vi "Buffer Overflow.vi"() -> ()   [LabVIEW 2010]
uses:
  <vilib>/express/express analysis/Spectral/XNode/ExpressSpectralMeasurementsBlockNode.xnode
  Instance           2 23Saved   Buffer Overflow .vi
  Instance           5 23Saved   Buffer Overflow .vi
  Instance           4 23Saved   Buffer Overflow .vi
  <vilib>/express/express analysis/Spectral/Block/exnSpectralBlock spectral measurements power poly.vi
  <vilib>/express/express analysis/Spectral/Block/exnSpectralBlock spectral measurements power DDT.vi
  Program Files/National Instruments/LabVIEW 2010/resource/objmgr/daqmx.rc
panel:
  out "주파수":dbl
  out "파워 스펙트럼":dynamicdata(graph)
  out "시간 데이터":dynamicdata(graph)
  out "DAQ 버퍼 크기":u32
  in  "정지":bool
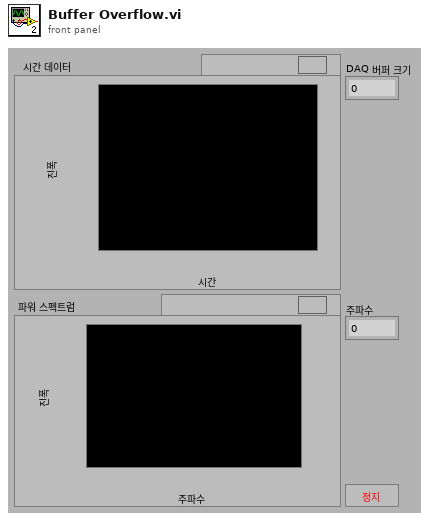
[diagram p1: front panel]
types:
  T1 = cluster{"averaging mode":u16, "weighting mode":u16, "number of averages":u32}
  T2 = cluster{"dB On (F)":bool, "unwrap phase (F)":bool, "convert to degree (F)":bool}
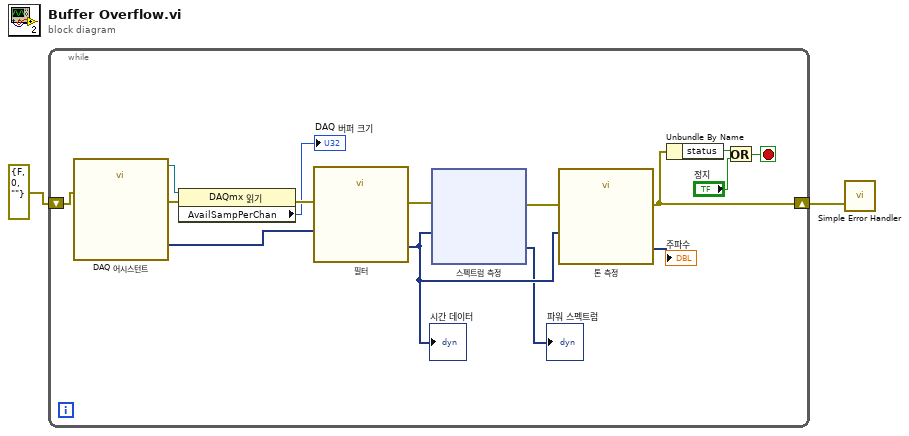
[diagram p0: block diagram]
diagram:
  n1 = while {
    shift-right: [w3] -> w2
    shift-left: errorcluster {"status"=FALSE, "code"=0, "source"=""} ("error out") -> [w13]
    stop <- w15 stop-if-true
    n2 = call "DAQ 어시스턴트"("error in"=w13) -> ("task out"=w14:refnum<k21>, "data"=w6:dynamicdata, "error out"=w12:errorcluster)  [unwired: 15 in, 1 out]
    n3 = property class="DAQmx 읽기"(reference=w14, error in=w12) -> (error out=w5:errorcluster, "AvailSampPerChan"=→"DAQ 버퍼 크기":u32)  [unwired: 1 out]
    n4 = call "필터"("error in (no error)"=w5, "Signal"=w6) -> ("error out"=w11:errorcluster, "Filtered Signal"=w10:dynamicdata)  [unwired: 8 in]
    "시간 데이터" <- w10
    n5 = xnode "스펙트럼 측정"("신호"=w10, "에러 입력(에러 없음)"=w11) -> ("파워 스펙트럼"=→"파워 스펙트럼":dynamicdata, "에러 출력"=w7:errorcluster)
    n6 = call "톤 측정"("error in (no error)"=w7, "Signals"=w10) -> ("error out"=w3:errorcluster, "Frequency"=→"주파수":dynamicdata)  [unwired: 8 in]
    n7 = Unbundle By Name(w3) -> ("status"=w17:bool)
    n8 = Or(x=w17, y="정지") -> (x .or. y?=w15:bool)
  }
  n9 = call <vilib>:"Simple Error Handler.vi"("error in (no error)"=w2) -> ()  [unwired: 4 in, 5 out]
